vi "LSX Set Prio Handler Pos.vi"(8 "error in (no error)":errorcluster, 10 "php":i32, 11 "lLSID":i32) -> (0 "error out":errorcluster, 3 "function return":i32)   [LabVIEW 2018, in "Tango.lvlib"]
doc: "TANGOAPI int TANGOCALL LSX_SetPrioHandlerPos (int lLSID, int php);"
uses:
  Tango.lvlib
  SubVIs/Tango_DLL.dll
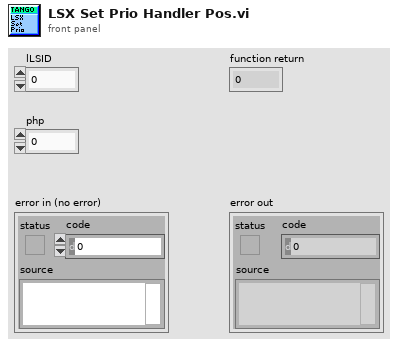
[diagram p1: front panel]
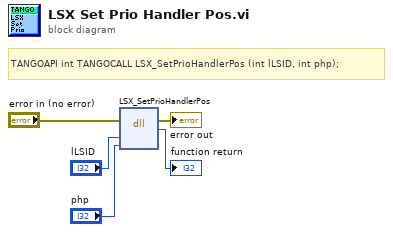
[diagram p0: block diagram]
diagram:
  # "TANGOAPI int TANGOCALL LSX_SetPrioHandlerPos (int lLSID, int php);"
  n1 = dll-call lib="C:/Users/Familie/Documents/LabviewIX81/lib/TANGO Stage/SubVIs/Tango_DLL.*" fn="LSX_SetPrioHandlerPos"(error in="error in (no error)", "lLSID"="lLSID", "php"="php") -> (error out=→"error out":errorcluster, →"function return":i32)  [unwired: 4 in, 1 out]
